vi "FSK_RECV_TEST.vi"() -> ()   [LabVIEW 2015]
uses:
  <vilib>/Utility/error.llb/DialogType.ctl
  <instrlib>/niUSRP/niUSRP Fetch Rx Data (CDB WDT).vi
panel:
  in  "数据源文件":path=path "C:/Users/admin/Desktop/USRP0902/USRP/Fsk/SendBit.mat"
  in  "接收码元速率":dbl=10000.0
  in  "信源比特长度":dbl=1000.0
  out "波形图":dbl[](graph)
  in  "Stop Button":bool
  in  "天线选择":string="RX2"
  out "实际接收增益":dbl=10.0 format="%#_6f"
  out "实际载波频率":dbl=1000000000.0 format="%#_6p"
  out "实际基带采样率":dbl=200000.0 format="%#_6p"
  in  "设定接收增益":dbl=10.0 format="%#_6f"
  in  "设定载波频率":dbl=1000000000.0 format="%#_6p"
  in  "设定基带采样率":dbl=200000.0 format="%#_6p"
  in  "设备IP":refnum<k15>="192.168.10.2"
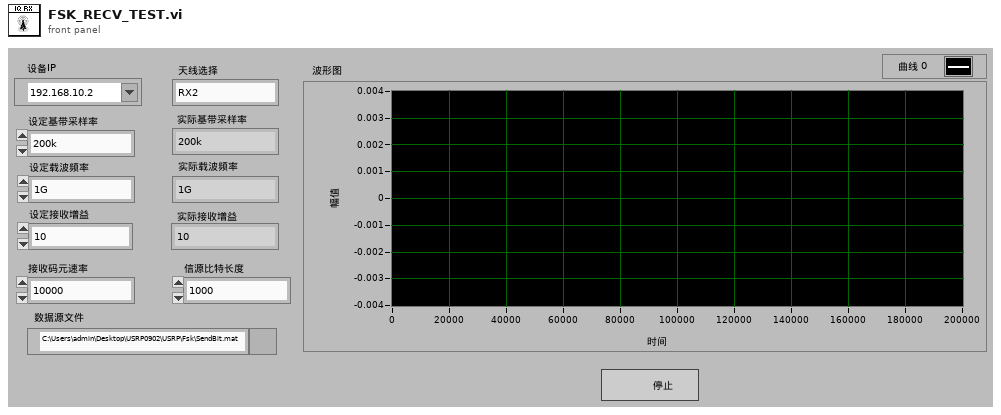
[diagram p1: front panel]
types:
  T1 = typedef "DialogType.ctl" = u16
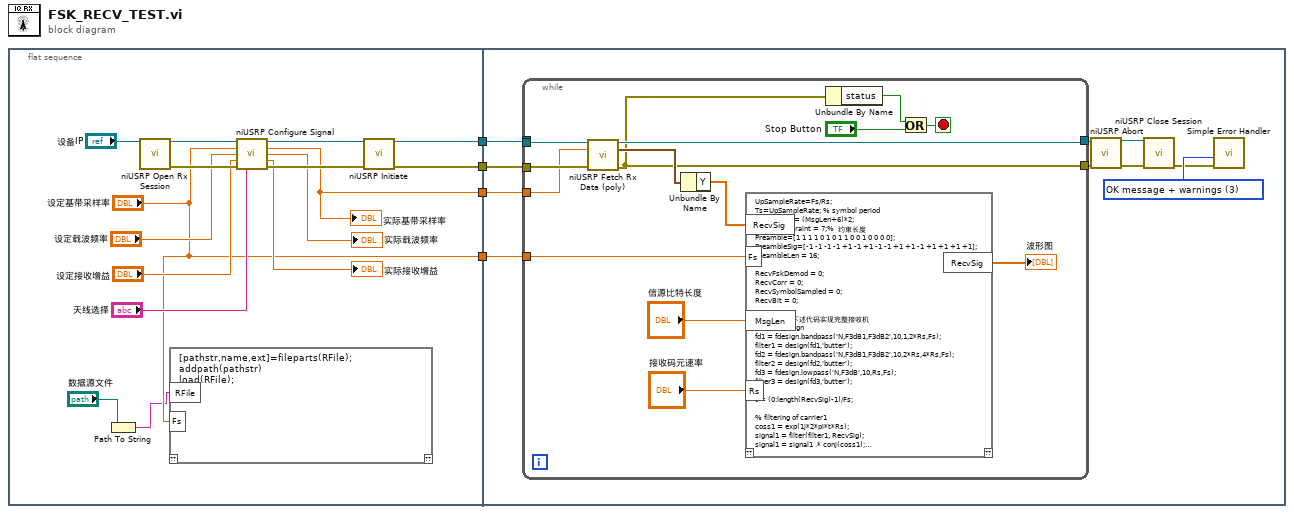
[diagram p0: block diagram]
diagram:
  n1 = flat-sequence {
    tunnel: [w11] -> w4
    tunnel: [w10] -> w3
    tunnel: ["设定基带采样率"] -> w2
    tunnel: [w9] -> w1
    tunnel: w4 -> [w26]
    tunnel: w3 -> [w25]
    tunnel: w2 -> [w22]
    tunnel: w1 -> [w21]
    frame #0 {
      n2 = Path To String(path="数据源文件") -> (string=w5:string)
      n3 = call <instrlib>:"niUSRP Open Rx Session.vi"("device names"="设备IP") -> ("session handle out"=w20:refnum<k15>, "error out"=w19:errorcluster)  [unwired: 13 in]
      n4 = script code="[pathstr,name,ext]=fileparts(RFile);\naddpath(pathstr)\nload(RFile);"("RFile"=w5, "Fs"="设定基带采样率") -> ()  [unwired: 2 out]
      n5 = call <instrlib>:"niUSRP Configure Signal.vi"("session handle"=w20, "IQ rate"="设定基带采样率", "carrier frequency"="设定载波频率", "gain"="设定接收增益", "error in (no error)"=w19, "active antenna"="天线选择") -> ("session handle out"=w14:refnum<k15>, "coerced IQ rate"=w9:dbl, "coerced carrier frequency"=→"实际载波频率":dbl, "coerced gain"=→"实际接收增益":dbl, "error out"=w16:errorcluster)  [unwired: 5 in]
      "实际基带采样率" <- w9
      n6 = call <instrlib>:"niUSRP Initiate.vi"("session handle"=w14, "error in (no error)"=w16) -> ("session handle out"=w11:refnum<k15>, "error out"=w10:errorcluster)  [unwired: 12 in]
    }
    frame #1 {
      w24 = T1 3 items=["no dialog", "OK message", "continue or stop message", "OK message + warnings", "continue/stop + warnings"] ("type of dialog (OK msg:1)")
      n7 = while {
        tunnel: [w38] -> _
        tunnel: [w43] -> w28
        tunnel: [w39] -> w27
        tunnel: w26 -> [w38]
        tunnel: w25 -> [w37]
        tunnel: w22 -> [w36]
        tunnel: w21 -> [w33]
        stop <- w42 stop-if-true
        n8 = call-poly <instrlib>:"niUSRP Fetch Rx Data (poly).vi"("session handle"=w38, "number of samples"=w33, "error in (no error)"=w37) -> ("session handle out"=w43:refnum<k15>, "data"=w40:waveform(cdb), "error out"=w39:errorcluster)  [unwired: 9 in, 1 out]
        n9 = Unbundle By Name ("Get Waveform Components")(w40) -> ("Y"=w35:cdb[])
        n10 = script code="UpSampleRate=Fs/Rs;\nTs=UpSampleRate; % symbol period\nSymbolLen = (MsgLen+6)*2;\nCoderConstraint = 7;%  约束长度 \nPreamble=[1 1 1 1 0 1 0 1 1 0 0 1 0 0 0 0];\nPreambleSig=[-1 -1 -1 -1 +1 -1 +1 -1 -1 +1 +1 -1 +1 +1 +1 +1];\nPreambleLen = 16;\n\nRecvFskDemod = 0;\nRecvCorr = 0;\nRecvSymbolSampled = 0;\nRecvBit = 0;\n\n%% 请完成下述代码实现完整接收机\n% filter design\nfd1 = fdesign.bandpass('N,F3dB1,F3dB2',10,1,2*Rs,Fs);\nfilter1 = design(fd1,'butter');\nfd2 = fdesign.bandpass('N,F3dB1,F3dB2',10,2*Rs,4*Rs,Fs);\nfilter2 = design(fd2,'butter');\nfd3 = fdesign.lowpass('N,F3dB',10,Rs,Fs);\nfilter3 = design(fd3,'butter');\n\nt = (0:length(RecvSig)-1)/Fs;\n\n% filtering of carrier1\ncoss1 = exp(1j*2*pi*t*Rs);\nsignal1 = filter(filter1, RecvSig);\nsignal1 = signal1 .* conj(coss1);\nsignal1 = filter(filter3, signal1);\n\n% filtering of carrier2\ncoss2 = exp(1j*2*pi*t*3*Rs);\nsignal2 = filter(filter2, RecvSig);\nsignal2 = signal2 .* conj(coss2);\nsignal2 = filter(filter3, signal2);\n\n% FSK demodulation\nRecvFskDemod = abs(signal1) - abs(signal2);%取长度\n\n% preamble search\nRecvCorr = zeros(1,floor(length(RecvFskDemod)/3));\nfor k=1:length(RecvFskDemod)/3 \n    RecvCorr(k) = sum(RecvFskDemod(k:Ts:k+PreambleLen*Ts-1).*PreambleSig);\nend\nRecvCorr = abs(RecvCorr);\n\n% sampled symbol\n[peak, pos] = max(RecvCorr);\nRecvSymbolSampled = RecvFskDemod(pos:Ts:pos+(PreambleLen+SymbolLen)*Ts-1);\nRecvSymbolSampled = real(sign(RecvSymbolSampled(PreambleLen+1:end)));\n\n% convolutoinal decoding\nsampled_code = round(max(RecvSymbolSampled,0));%round((1-RecvSymbolSampled)/2);\nt = poly2trellis(CoderConstraint, [171, 133]);\ntb = 2;\ndecoded = vitdec(sampled_code,t,tb,'trunc','hard');\nRecvBit = decoded(1:end-6);\nfigure;plot(abs(RecvBit-SendBit));title('abs(RecvBit-SendBit)：接收发送比特错误');"("RecvSig"=w35, "Fs"=w36, "MsgLen"="信源比特长度", "Rs"="接收码元速率") -> ("RecvSig"=→"波形图":cdb[])  [unwired: 2 out]
        n11 = Unbundle By Name(w39) -> ("status"=w44:bool)
        n12 = Or(x=w44, y="Stop Button") -> (x .or. y?=w42:bool)
      }
      n13 = call <instrlib>:"niUSRP Abort.vi"("session handle"=w28, "error in (no error)"=w27) -> ("session handle out"=w30:refnum<k15>, "error out"=w29:errorcluster)  [unwired: 12 in]
      n14 = call <instrlib>:"niUSRP Close Session.vi"("session handle"=w30, "error in (no error)"=w29) -> ("error out"=w23:errorcluster)  [unwired: 13 in]
      n15 = call <vilib>:"Simple Error Handler.vi"("type of dialog (OK msg:1)"=w24, "error in (no error)"=w23) -> ()  [unwired: 3 in, 5 out]
    }
  }
